vi "TriggerDetectorWithAutorearming.vi"() -> ()   [LabVIEW 2013]
panel:
  in  "TriggerAutoReArm":i32=-1
  out "TriggerArmed":bool
  in  "FireTrigger":bool
  in  "ArmTrigger":bool
  out "TriggerFired":bool
  in  "ResetTrigger":bool
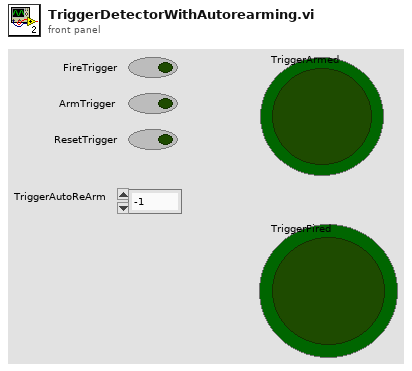
[diagram p1: front panel]
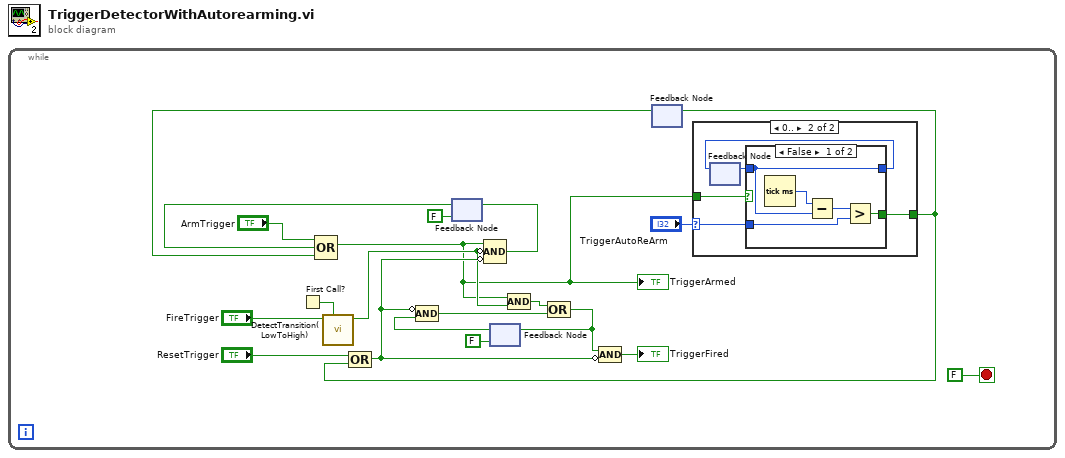
[diagram p0: block diagram]
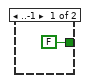
[diagram p2: hidden frame]
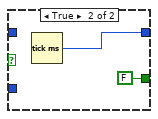
[diagram p3: hidden frame]
diagram:
  n1 = while {
    stop <- FALSE stop-if-true
    n2 = First Call?() -> (First Call?: T/F=w4:bool)
    n3 = call "DetectTransition(LowToHigh).vi"("First Call?: T/F"=w4, "InputSignal"="FireTrigger") -> ("RaisingFrontDetected"=w3:bool)  [unwired: 9 in]
    n4 = feedback #1(FALSE) -> (w18:bool)
    n5 = feedback #2(FALSE) -> (w11:bool)
    n6 = feedback #3() -> (w8:bool)  [unwired: 1 in]
    n7 = Compound Arithmetic op=OR("ArmTrigger", w18, w8) -> (w2:bool)
    "TriggerArmed" <- w2
    n8 = Compound Arithmetic op=AND(w2, w3) -> (w9:bool)
    n9 = case shown="0.." "TriggerAutoReArm" {
      selector: "TriggerAutoReArm" -> [_ w23]
      tunnel: [FALSE w22] -> w1
      tunnel: w2 -> [_ w24]
      frame ..-1 {
      }
      frame 0.. {
        n10 = feedback #4() -> (w25:u32)  [unwired: 1 in]
        n11 = case shown="False" w24 {
          tunnel: [w30 w33] -> w26
          tunnel: w25 -> [w30 _]
          tunnel: w23 -> [w28 _]
          tunnel: [w27 FALSE] -> w22
          frame False {
            n12 = Tick Count (ms)() -> (millisecond timer value=w31:u32)
            n13 = Subtract(x=w31, y=w30) -> (x-y=w29:u32)
            n14 = Greater?(x=w29, y=w28) -> (0:w27:bool)
          }
          frame True {
            n15 = Tick Count (ms)() -> (millisecond timer value=w33:u32)
          }
        }
        n16 = feedback-in #4(w26) -> ()
      }
    }
    n17 = Compound Arithmetic op=OR("ResetTrigger", w1) -> (w6:bool)
    n18 = Compound Arithmetic op=AND(invert w6, w11) -> (w12:bool)
    n19 = Compound Arithmetic op=AND(w2, invert w3, invert w6) -> (w17:bool)
    n20 = feedback-in #1(w17) -> ()
    n21 = Compound Arithmetic op=OR(w9, w12) -> (w14:bool)
    n22 = feedback-in #2(w14) -> ()
    n23 = Compound Arithmetic op=AND(w14, invert w6) -> (→"TriggerFired":bool)
    n24 = feedback-in #3(w1) -> ()
  }
